vi "plot da wedge.vi"() -> ()   [LabVIEW 2010]
uses:
  <vilib>/picture/3D Picture Control/NI_3D Picture Control.lvlib
panel:
  out "Boolean":bool
  in  "Skip cleanup?":bool
  in  "System Save Button":bool
  in  "Grain Growth and Geometry":T1={"Min Grain Length (A)"=12.0, "Min Angle from GB plane"=15.0, "GB Overlap Length (A)"=0.0}
  in  "Collision Removal":T2={"Min Seperation Distance (A)"=2.0, "Edge Duplication Range (A)"=3.0}
  in  "Co-incident Tolerance":dbl=0.05
  in  "Options":cluster{"Border?":bool, "Bonds?":bool}
  out "Grain Boundary":T3={"Structure Name"="(0.00) twist [1.000,0.602,0.030] [1.000,0.731,0.221] (0.00,0.00,0.00)T GB", "Lattice vector a"=[270.03, 0.0, 0.0], "Lattice vector b"=[0.0, 270.03, 0.0], "Lattice vector c"=[0.0, 0.0, 6.006], "Atoms Array"=[{"Atom Name"="Cd", "Positions (Direct)"=array6055x3[18165 elements], "Positions (Cartesian)"=array6055x3[18165 elements]}, {"Atom Name"="Te", "Positions (Direct)"=array6080x3[18240 elements], "Positions (Cartesian)"=array6080x3[18240 elements]}], "# of atoms"=12135} {"Atoms Array"."Positions (Cartesian)" format="%#_4f"; "Atoms Array"."Positions (Direct)" format="%#_4f"}
  in  "Vesta .exe Location":path=path "C:/Program Files (x86)/VESTA/VESTA.exe"
  in  "Grain Boundary Definition":T4={"Grain 1 Orientation"=[1.0, 1.0, 0.0], "Grain 2 Orientation"=[1.0, 1.0, 1.0], "Twist Angle (Deg)"=0.0, "Translation Vector"=[0.0, 0.0, 0.0]}
  out "Object with atoms":refnum<vi>
  in  "Load G2 VESTA":bool
  out "Grain Boundary Render":refnum<vi>(3d-picture)
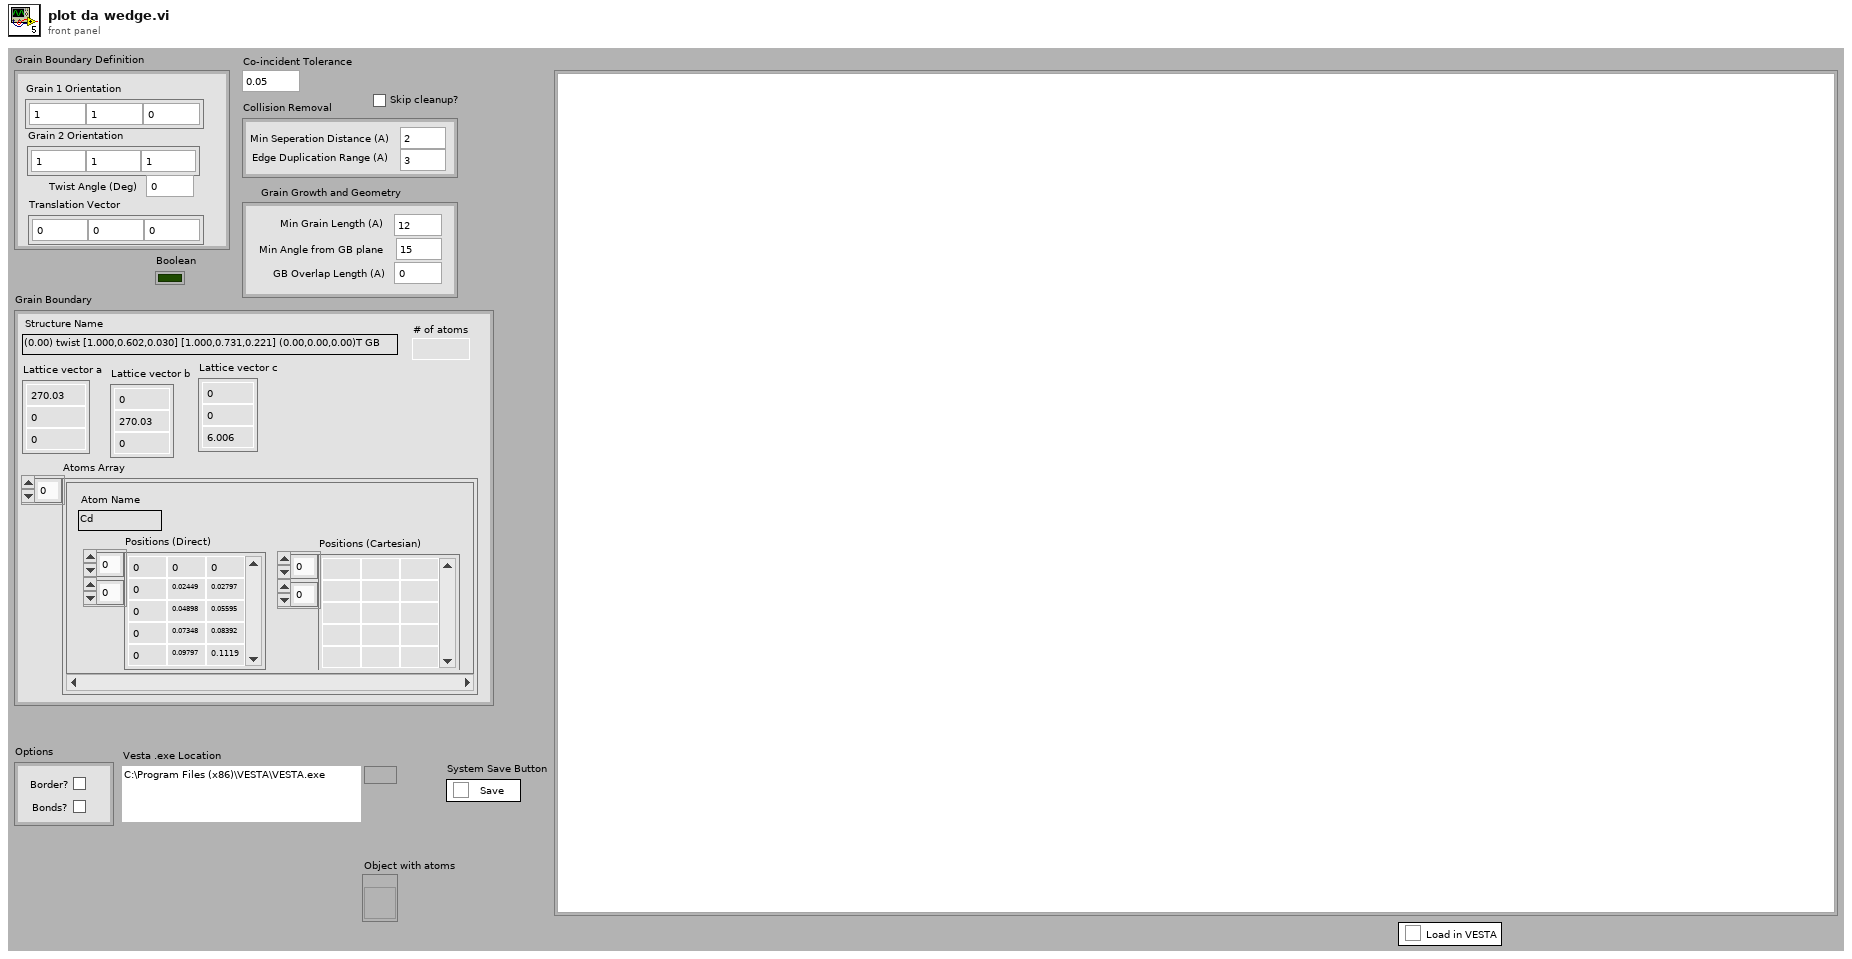
[diagram p1: front panel]
types:
  T1 = cluster{"Min Grain Length (A)":dbl, "Min Angle from GB plane":dbl, "GB Overlap Length (A)":dbl}
  T2 = cluster{"Min Seperation Distance (A)":dbl, "Edge Duplication Range (A)":dbl}
  T3 = cluster{"Structure Name":string, "Lattice vector a":dbl[], "Lattice vector b":dbl[], "Lattice vector c":dbl[], "Atoms Array":cluster{"Atom Name":string, "Positions (Direct)":dbl[][], "Positions (Cartesian)":dbl[][]}[], "# of atoms":i32}
  T4 = cluster{"Grain 1 Orientation":dbl[], "Grain 2 Orientation":dbl[], "Twist Angle (Deg)":dbl, "Translation Vector":dbl[]}
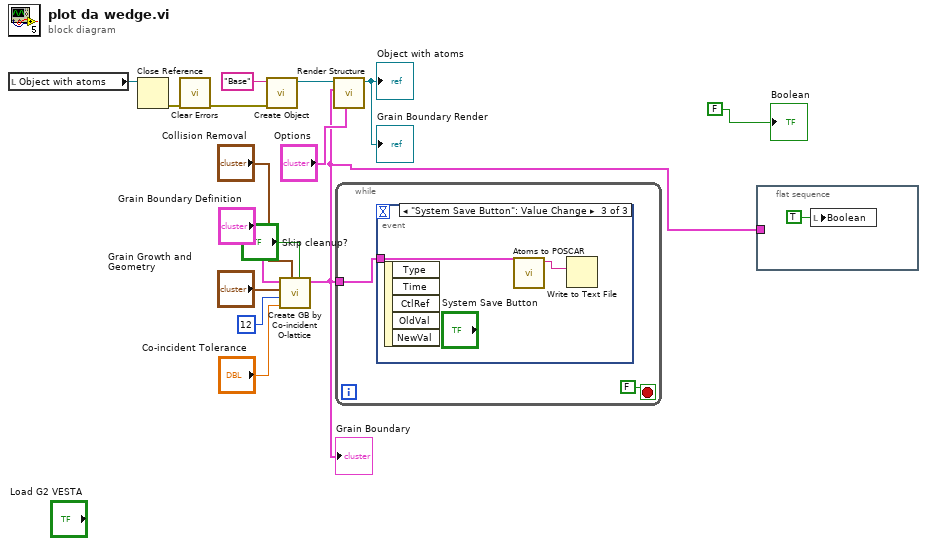
[diagram p0: block diagram]
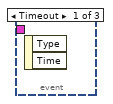
[diagram p2: hidden frame]
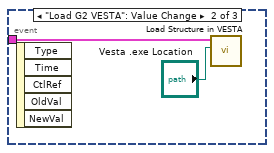
[diagram p3: hidden frame]
diagram:
  n1 = local read "Object with atoms"() -> (w12:refnum<vi>)
  n2 = Close Reference(reference=w12) -> (error out=w10:errorcluster)  [unwired: 1 in]
  n3 = call <vilib>:"Clear Errors.vi"("error in (no error)"=w10) -> ("error out"=w9:errorcluster)  [unwired: 6 in]
  n4 = call <vilib>:"Create Object.vi"("error in (no error)"=w9, "Name"="Base") -> ("Scene:New Object"=w13:refnum<vi>)  [unwired: 9 out]
  n5 = call "Create GB by Co-incident O-lattice.vi"("Skip cleanup?"="Skip cleanup?", "Collision Removal"="Collision Removal", "Co-incident Tolerance"="Co-incident Tolerance", "Number of integers to search"=12, "Grain Growth and Geometry"="Grain Growth and Geometry", "Grain Boundary Definition"="Grain Boundary Definition") -> ("Grain Boundary"=w1:T3)  [unwired: 3 in, 2 out]
  "Grain Boundary" <- w1
  n6 = call "Render Structure.vi"("Options"="Options", "Atomic Structure"=w1, "Base Object"=w13) -> ("Object with atoms"=→"Grain Boundary Render" →"Object with atoms":refnum<vi>)  [unwired: 8 in]
  n7 = while {
    tunnel: w1 -> [w16]
    stop <- FALSE stop-if-true
    n8 = event shown="[2] \"System Save Button\": Value Change" {
      selector: _ -> [_ _ _]
      dyn-events: _ -> [_ _ _]
      timeout: _ -> [_ _ _]
      tunnel: w16 -> [_ w18 w21]
      event Timeout {
        n9 = event-data() -> ()  [unwired: 1 in, 2 out]
      }
      event "Load G2 VESTA": Value Change {
        n10 = event-data() -> ()  [unwired: 1 in, 5 out]
        n11 = call "Load Structure in VESTA.vi"("Vesta .exe Location"="Vesta .exe Location", "Atomic Structure"=w18) -> ()  [unwired: 10 in]
      }
      event "System Save Button": Value Change {
        n12 = event-data() -> ()  [unwired: 1 in, 5 out]
        n13 = call "Atoms to POSCAR.vi"("Atomic Structure"=w21) -> ("POSCAR File"=w20:string)  [unwired: 10 in]
        n14 = Write to Text File(text=w20) -> ()  [unwired: 3 in, 3 out]
      }
    }
  }
  n15 = flat-sequence {
    tunnel: w1 -> [_]
    frame #0 {
      n16 = local write "Boolean"(TRUE ("Boolean")) -> ()
    }
  }
  "Boolean" <- FALSE
